vi "Assert Windows Bounds.vi"(6 "VI reference":refnum<vi>, 7 "Test Description":string, 8 "error in":errorcluster, 10 "Expected Position":T1, 11 "Editor Position in":refnum<class "Editor Position.lvclass">) -> (0 "error out":errorcluster, 3 "Editor Position out":refnum<class "Editor Position.lvclass">)   [LabVIEW 2020, in "Editor Position.lvclass"]
doc: "Gets the current window bounds and asserts the unit test."
uses:
  Editor Position.lvclass
  Editor Position.lvclass/Editor Position.ctl
  94d62f03-ad9e-4251-b5e0-ea12bf9f98d6.vi
  <vilib>/Utility/miscctls.llb/LVRectTypeDef.ctl
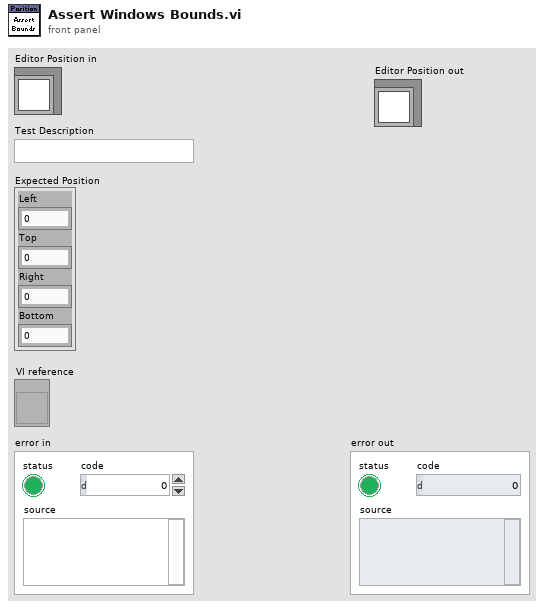
[diagram p1: front panel]
types:
  T1 = typedef "LVRectTypeDef.ctl" = cluster{"Left":i16, "Top":i16, "Right":i16, "Bottom":i16}
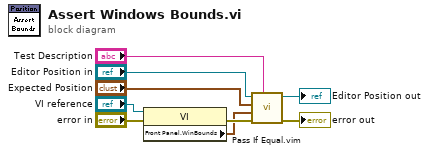
[diagram p0: block diagram]
diagram:
  n1 = property class="VI"(reference="VI reference", error in="error in") -> (error out=w9:errorcluster, "Front Panel.WinBounds"=w4:T1)  [unwired: 1 out]
  n2 = call "Pass If Equal.vim"("Description"="Test Description", "error in (no error)"=w9, "Actual"=w4, "Expected"="Expected Position", "LUnit Test Case In"="Editor Position in") -> ("error out"=→"error out":errorcluster, "LUnit Test Case Out"=→"Editor Position out":refnum<class "Editor Position.lvclass">)  [unwired: 5 in]
